vi "ITC503 Control Panel.vi"(8 "error in (no error)":errorcluster, 11 "Class":refnum<class "ITC 503.lvclass">) -> (0 "error out":errorcluster, 3 "ITC 503 out":refnum<class "ITC 503.lvclass">)   [LabVIEW 2015, in "ITC 503.lvclass"]
uses:
  ITC 503.lvclass
  Controls/ITC503 FP Data.ctl
panel:
  in  "Data":T1={"Channels to measure"=[1]}
  # "1-3: sensors\n6: heater V\n7: gas flow\n\nmore in ITC manual"
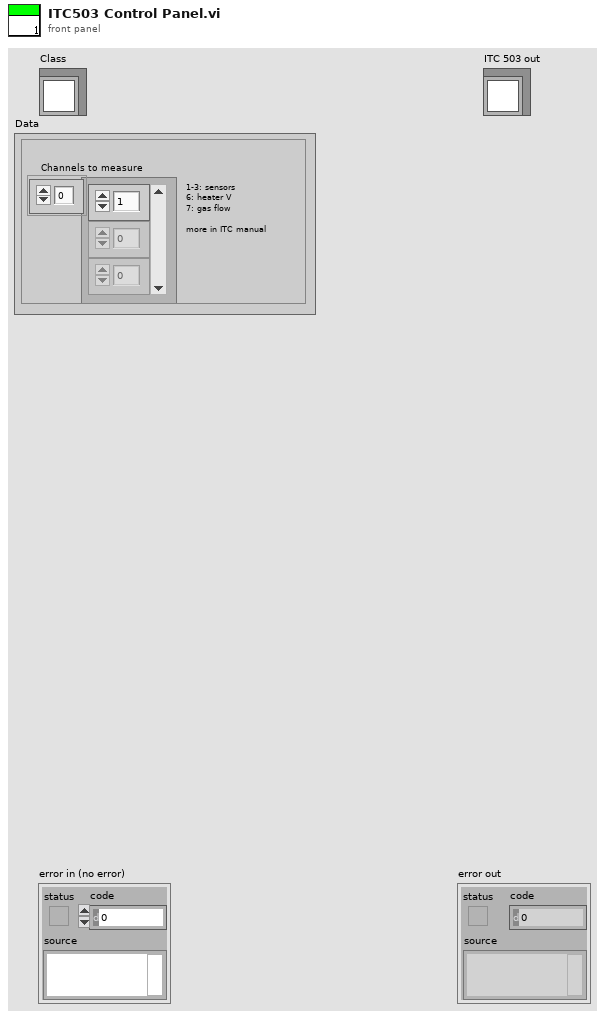
[diagram p1: front panel]
types:
  T1 = typedef "ITC503 FP Data.ctl" = cluster{"Channels to measure":i32[]}
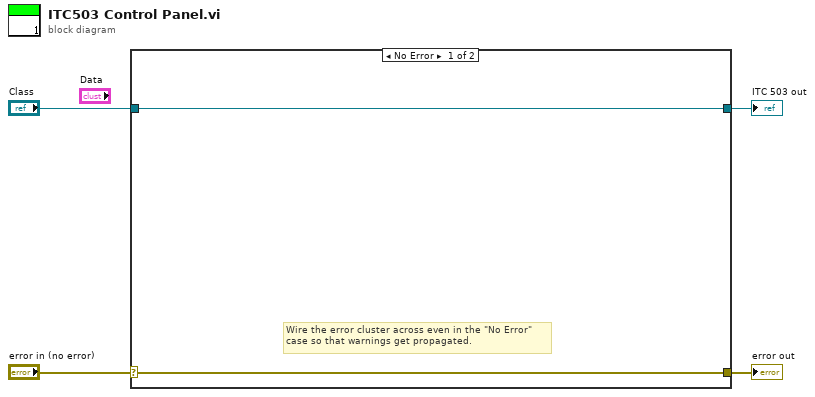
[diagram p0: block diagram]
diagram:
  n1 = case shown="No Error" "error in (no error)" {
    selector: "error in (no error)" -> [w5 w8]
    tunnel: [w5 w8] -> w3
    tunnel: [w6 w7] -> w1
    tunnel: "Class" -> [w6 w7]
    frame No Error {
      # "Wire the error cluster across even in the \"No Error\"\ncase so that warnings get propagated."
    }
    frame Error {
    }
  }
  "error out" <- w3
  "ITC 503 out" <- w1
